vi "FPGA cRIOMain_v9.vi"() -> ()   [LabVIEW 2019]
uses:
  TypeDefs/AO mode TabCtrl.ctl
  TypeDefs/SamplingModeEnum.ctl
  TypeDefs/AI_channelEnum.ctl
  <vilib>/Platform/TimedLoop/XDataNode/timing_clust.ctl
  <vilib>/Platform/TimedLoop/XDataNode/nitl_modes.ctl
  <vilib>/Platform/TimedLoop/XDataNode/wakeup.ctl
  <vilib>/rvi/Emulation/niFpgaGetClockAttributes.vi
  <vilib>/rvi/Emulation/niFpgaSctlEmulationGetInTimedLoop.vi
  <vilib>/rvi/Emulation/niFpgaEmulationReportErrorSimple.vi
  <vilib>/rvi/eio/common/nirviEmuTemplateMethod_errors.vi
  <vilib>/rvi/Emulation/niFpgaEmulationIsFPGAContextNoSignature.vi
  <vilib>/rvi/errors/niFpgaSetErrorForExecOnDevCompSimple.vi
  <vilib>/rvi/eio/common/nirviEmuReportErrorAndStop.vi
  <vilib>/rvi/DataTransferAndStorage/Container/Common/niFpgaContainerGetUniqueNameForEmu.vi
  <vilib>/rvi/FIFO/Fifo_Resource/nirvififoEmulationSetSize.vi
  <vilib>/rvi/FIFO/Fifo_Resource/nirviFifoEmulationQueueMgr.vi
  <instcachedir>/0/nirviFifoEmulationQueueMgr_E5CAEC123FF24DC58D834DCA3CDAA9B5.lvgen/nirviFifoEmulationQueueMgr_E5CAEC123FF24DC58D834DCA3CDAA9B5_000.vi
  <vilib>/rvi/FIFO/Fifo_Resource/nirvififoEmulationDetermineInputValidOut.vi
  <vilib>/rvi/FIFO/Fifo_Resource/nirvififoEmulationCreateLock.vi
  <vilib>/rvi/Emulation/niFpgaProcessEmulError.vi
  <vilib>/rvi/FIFO/Fifo_Resource/nirvififoEmulationObtainLock.vi
  <vilib>/rvi/FIFO/Fifo_Resource/nirvififoEmulationReleaseLock.vi
  <vilib>/rvi/occurrence/nirviWaitOnOccurrenceBase.vi
  <vilib>/rvi/errors/nirviReportUnexpectedCaseInternalError.vi
  <vilib>/rvi/errors/nirviReportUnexpectedCaseInternalError (U32).vi
  <vilib>/rvi/Emulation/niFpgaCriticalErrorInLSC.vi
  <instcachedir>/0/nirviFifoEmulationQueueMgr_E5CAEC123FF24DC58D834DCA3CDAA9B5.lvgen/nirviFifoEmulationQueueMgr_E5CAEC123FF24DC58D834DCA3CDAA9B5_006.vi
  <vilib>/Utility/error.llb/Clear Errors.vi
  <vilib>/rvi/Memory/Memory_Emulation/niFpgaMemoryEmulationCacheClearOnFirstRun.vi
  <vilib>/rvi/Memory/Memory_Emulation/nirvimemoryEmulationManagerCache_MakeExclusive.vi
  <vilib>/rvi/Memory/Memory_Emulation/niFpgaMemoryEmulationValidateCache.vi
  <vilib>/rvi/Memory/Memory_Emulation/nirvimemoryEmulationManagerCache_InsertValue.vi
  <vilib>/rvi/Memory/Memory_Emulation/nirvimemoryEmulationManagerCache_ReleaseExclusive.vi
  <vilib>/rvi/Memory/Memory_Emulation/nirvimemoryEmulationManagerCache_GetValue.vi
  <vilib>/rvi/Memory/Memory_Emulation/nirvimemoryEmulationManagerCache_SetValue.vi
  <vilib>/rvi/Analysis/common/codeGenErrors/XNode/niFpgaXNodeCodeGenErrorHandle.vi
  <instcachedir>/0/nirviFifoEmulationQueueMgr_E5CAEC123FF24DC58D834DCA3CDAA9B5.lvgen/nirviFifoEmulationQueueMgr_E5CAEC123FF24DC58D834DCA3CDAA9B5_015.vi
  <vilib>/eio/EIONode/EIONode.xnode
  <vilib>/rvi/DataTransferAndStorage/Container/XNode/niFpgaContainer.xnode
  <vilib>/rvi/FIFO/Fifo_Resource/nirvififoEmulationWrite.vi
  <vilib>/rvi/FIFO/Fifo_Resource/nirvififoEmulationRead.vi
  <vilib>/rvi/DataTransferAndStorage/Register/Emulation/niFpgaRegisterEmulation.vi
  <vilib>/rvi/FXPMathLib/FxpMul/XNode/nifxpmath_Multiplier.xnode
  <vilib>/rvi/Analysis/measure/LMRsmpl/XNode/niFPGA Rational Resampler.xnode
  <vilib>/Platform/TimedLoop/XDataNode/XDataNode.xnode
  <vilib>/Platform/TimedLoop/XDataNode/XDNodeRunTimeDep.lvlib
  <vilib>/rvi/FXPMathLib/sim/FxpSim.dll
panel:
  out "FPGA AI-M DMA\nOverflow?":bool
  out "AI M-2 loop time-2 [ticks]":u32
  out "AI M loop time [ticks]":u32
  out "FPGA AI DMA\nOverflow?":bool
  out "AI Processing\nLoop Rate to high?":bool
  in  "AI Process Time [ticks]":u32=125
  in  "Select Channel":T1
  out "Unable to\nsample at desired\nSample Rate?":bool
  out "Processing Loop time [ticks]":u32
  in  "Sampling Mode":T2
  in  "AO mode":T3
  in  "AO Out [V]":fxp<+/-,18,5> format="%#.6g"
  in  "AO enable?":bool
  out "AI In [V]":fxp<+/-,25,5> format="%#.6g"
  out "FPGA AO DMA\nOverflow?":bool
  out "Int. Output":fxp<+/-,20,5> format="%.17g"
  out "Raw AI Input":fxp<+/-,25,5> format="%.21g"
  in  "Sample Time [ticks]":u32=125
  out "AO Loop time [ticks]":u32
  out "AI Loop time [ticks]":u32
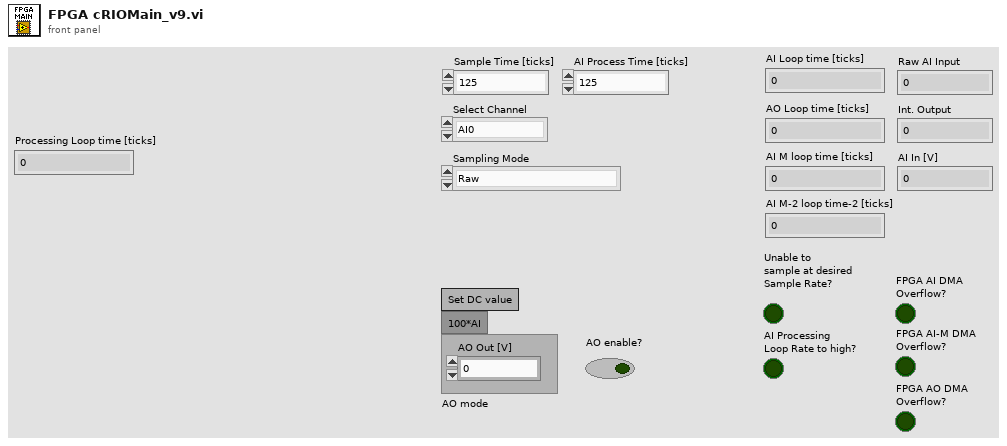
[diagram p1: front panel]
types:
  T1 = typedef "AI_channelEnum.ctl" = enum16{"AI0", "AI1", "AI2", "AI3"}
  T2 = typedef "SamplingModeEnum.ctl" = enum16{"Raw", "M64 (ReSpl)", "M128 (ReSpl)", "4pt MA (AI) + M64 (ReSpl)", "LPF (Proc.)", "4pt MA (AI) + LPF (Proc.)", "4pt MA (Proc.) + LPF (Proc.)"}
  T3 = typedef "AO mode TabCtrl.ctl" = enum32{"Set DC value", "100*AI"}
  T4 = typedef "XDNodeRunTimeDep.lvlib/timing_clust.ctl" = cluster{"Expected End [f-1]":u64, "Actual End [f-1]":u64, "Finished Late? [f-1]":bool, "Expected End [i-1]":u64, "Actual End [i-1]":u64, "Finished Late? [i-1]":bool, "Expected Start [i]":u64, "Actual Start [i]":u64, "Expected Start [f]":u64, "Actual Start [f]":u64, "Source Name":string, "Structure Name":string, "Period":i64, "Deadline":i64, "Offset":i64, "Start":i64, "Priority":i32, "Timeout":i32, "Mode":T5, "Wakeup Reason":T6, "Error":errorcluster, "Source Type":string, "Secondary Source Type":string, "Global End Time":u64, "Global Start Time":u64, "Frame Duration":u64, "Iteration Duration":u64, "Assigned CPU":i32, "I/O Scan Engine Mode":u32}
  T5 = typedef "XDNodeRunTimeDep.lvlib/nitl_modes.ctl" = enum32{"No Change", "Process missed periods, maintain original phase", "Discard missed periods, maintain original phase", "Process missed periods, ignore original phase", "Discard missed periods, ignore original phase"}
  T6 = typedef "XDNodeRunTimeDep.lvlib/wakeup.ctl" = enum32{"Normal", "Aborted", "Asynchronous wakeup", "Timing source error", "Timed loop error", "Timeout"}
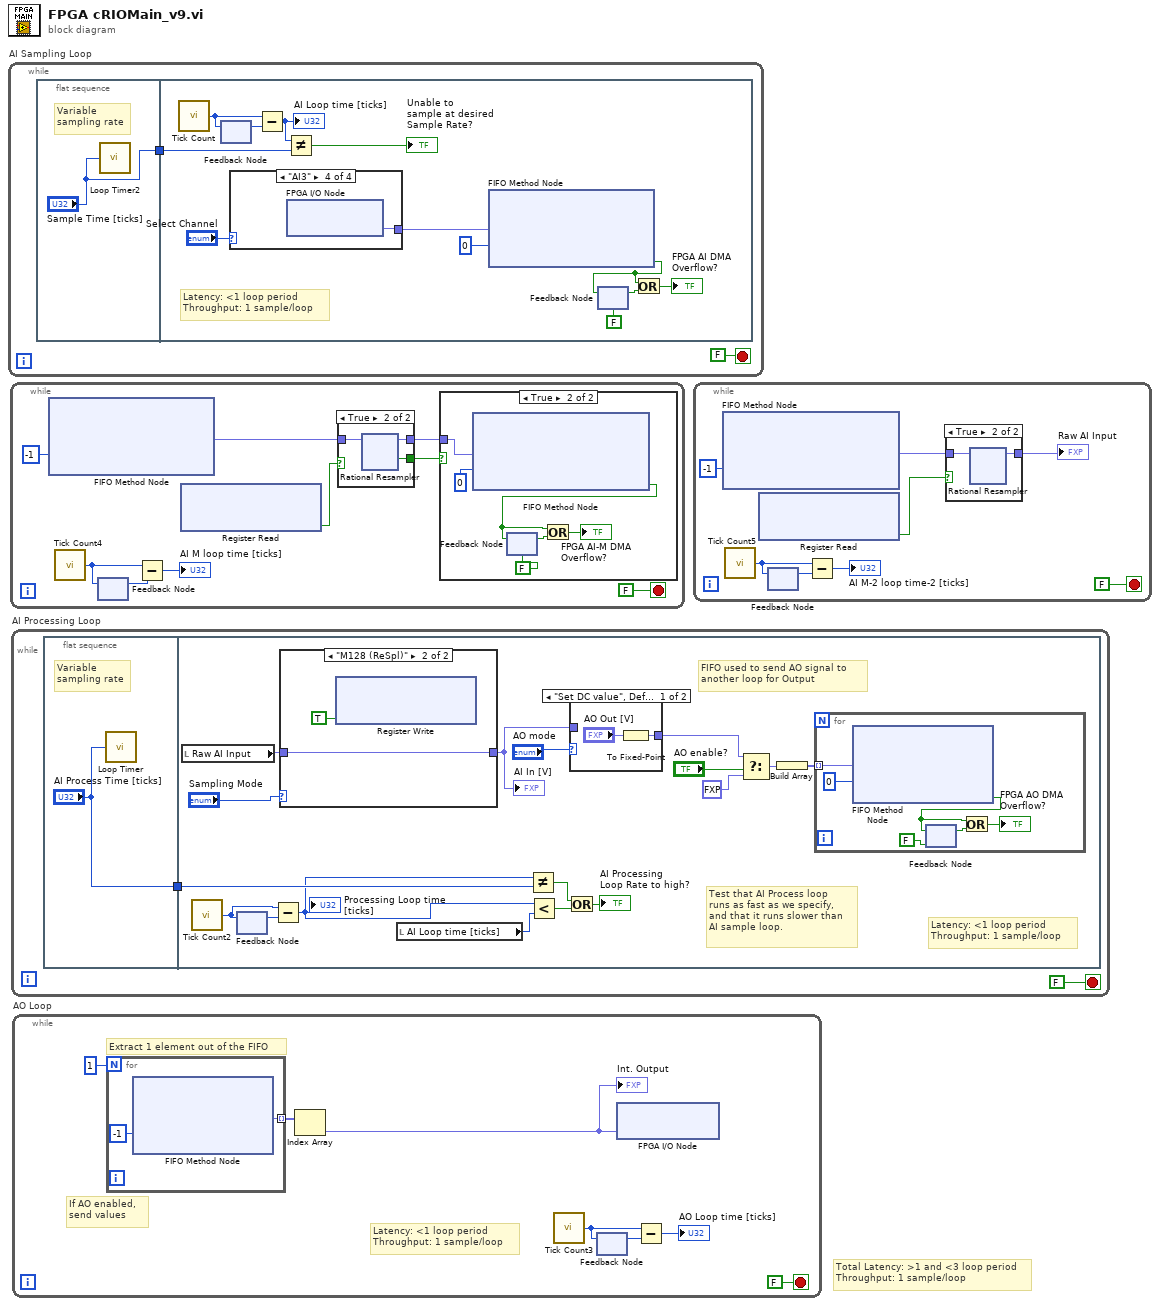
[diagram p0: block diagram]
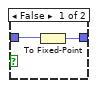
[diagram p2: hidden frame]
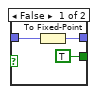
[diagram p4: hidden frame]
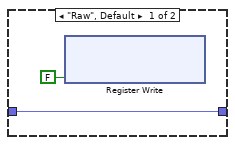
[diagram p5: hidden frame]
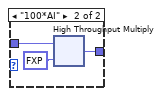
[diagram p6: hidden frame]
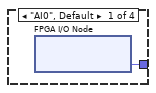
[diagram p7: hidden frame]
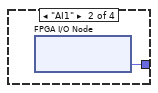
[diagram p8: hidden frame]
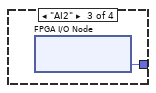
[diagram p9: hidden frame]
diagram:
  # "Total Latency: >1 and <3 loop period\nThroughput: 1 sample/loop"
  n1 = while "AI Sampling Loop" {
    stop <- FALSE stop-if-true
    n2 = flat-sequence {
      tunnel: ["Sample Time [ticks]"] -> w1
      tunnel: w1 -> [w12]
      frame #0 {
        # "Variable\nsampling rate"
        n3 = call "Loop Timer2"("Count(Ticks)"="Sample Time [ticks]") -> ()  [unwired: 1 out]
      }
      frame #1 {
        # "Latency: <1 loop period\nThroughput: 1 sample/loop"
        n4 = call "Tick Count"() -> ("Tick Count(Ticks)"=w15:u32)
        n5 = feedback #1() -> (w14:u32)  [unwired: 1 in]
        n6 = feedback-in #1(w15) -> ()
        n7 = case shown="\"AI3\"" "Select Channel" {
          tunnel: [w16 w17 w18 w19] -> w4
          frame "AI0", Default {
            n8 = xnode "FPGA I/O Node"() -> ("Mod4/AI0"=w16:fxp<+/-,24,5>)  [unwired: 1 in, 1 out]
          }
          frame "AI1" {
            n9 = xnode "FPGA I/O Node"() -> ("Mod4/AI1"=w17:fxp<+/-,24,5>)  [unwired: 1 in, 1 out]
          }
          frame "AI2" {
            n10 = xnode "FPGA I/O Node"() -> ("Mod4/AI2"=w18:fxp<+/-,24,5>)  [unwired: 1 in, 1 out]
          }
          frame "AI3" {
            n11 = xnode "FPGA I/O Node"() -> ("Mod4/AI3"=w19:fxp<+/-,24,5>)  [unwired: 1 in, 1 out]
          }
        }
        n12 = Subtract(x=w15, y=w14) -> (x-y=w13:u32)
        "AI Loop time [ticks]" <- w13
        n13 = Not Equal?(x=w13, y=w12) -> (x != y?=→"Unable to\nsample at desired\nSample Rate?":bool)
        n14 = xnode ("FIFO Method Node")("Element"=w4, "Timeout"=0) -> ("Timed Out?"=w7:bool)  [unwired: 1 in, 1 out]
        n15 = feedback #2(FALSE ("Timed Out?")) -> (w9:bool)
        n16 = feedback-in #2(w7) -> ()
        n17 = Or(x=w7, y=w9) -> (x .or. y?=→"FPGA AI DMA\nOverflow?":bool)
      }
    }
  }
  n18 = while {
    stop <- FALSE stop-if-true
    n19 = xnode ("FIFO Method Node")("Timeout"=-1) -> ("Element"=w22:fxp<+/-,24,5>)  [unwired: 1 in, 2 out]
    n20 = call "Tick Count4"() -> ("Tick Count(Ticks)"=w26:u32)
    n21 = feedback #3() -> (w25:u32)  [unwired: 1 in]
    n22 = feedback-in #3(w26) -> ()
    n23 = Subtract(x=w26, y=w25) -> (x-y=→"AI M loop time [ticks]":u32)
    n24 = xnode ("Register Read")() -> ("Data"=w23:bool)  [unwired: 1 in, 1 out]
    n25 = case shown="True" w23 {
      tunnel: w22 -> [w36 w40]
      tunnel: [w37 w39] -> w21
      tunnel: [TRUE ("output valid") w38] -> w20
      frame False {
        n26 = To Fixed-Point(number=w36) -> (fixed-point=w37:fxp<+/-,25,5>)  [unwired: 1 in]
      }
      frame True {
        n27 = xnode "Rational Resampler"("input data"=w40) -> ("output data"=w39:fxp<+/-,25,5>, "output valid"=w38:bool)  [unwired: 1 out]
      }
    }
    n28 = case shown="True" w20 {
      tunnel: w21 -> [_ w34]
      frame False {
      }
      frame True {
        n29 = xnode ("FIFO Method Node")("Element"=w34, "Timeout"=0) -> ("Timed Out?"=w29:bool)  [unwired: 1 in, 1 out]
        n30 = feedback #4(FALSE ("Timed Out?")) -> (w32:bool)
        n31 = feedback-in #4(w29) -> ()
        n32 = Or(x=w29, y=w32) -> (x .or. y?=→"FPGA AI-M DMA\nOverflow?":bool)
      }
    }
  }
  n33 = while "AI Processing Loop" {
    stop <- FALSE stop-if-true
    n34 = flat-sequence {
      tunnel: ["AI Process Time [ticks]"] -> w75
      tunnel: w75 -> [w79]
      frame #0 {
        # "Variable\nsampling rate"
        n35 = call "Loop Timer"("Count(Ticks)"="AI Process Time [ticks]") -> ()  [unwired: 1 out]
      }
      frame #1 {
        # "Test that AI Process loop\nruns as fast as we specify,\nand that it runs slower than \nAI sample loop."
        # "Latency: <1 loop period\nThroughput: 1 sample/loop"
        # "FIFO used to send AO signal to \nanother loop for Output"
        n36 = local read "Raw AI Input"() -> (w83:fxp<+/-,25,5>)
        n37 = call "Tick Count2"() -> ("Tick Count(Ticks)"=w93:u32)
        n38 = feedback #5() -> (w94:u32)  [unwired: 1 in]
        n39 = feedback-in #5(w93) -> ()
        n40 = Subtract(x=w93, y=w94) -> (x-y=w78:u32)
        "Processing Loop time [ticks]" <- w78
        n41 = case shown="\"M128 (ReSpl)\"" "Sampling Mode" {
          tunnel: [w95 w97] -> w91
          tunnel: w83 -> [w95 w97]
          frame "Raw", Default {
            n42 = xnode ("Register Write")("Data"=FALSE) -> ()  [unwired: 1 in, 1 out]
          }
          frame "M128 (ReSpl)" {
            n43 = xnode ("Register Write")("Data"=TRUE) -> ()  [unwired: 1 in, 1 out]
          }
        }
        "AI In [V]" <- w91
        n44 = local read "AI Loop time [ticks]"() -> (w84:u32)
        n45 = Not Equal?(x=w78, y=w79) -> (x != y?=w81:bool)
        n46 = Less?(x=w78, y=w84) -> (x < y?=w80:bool)
        n47 = Or(x=w81, y=w80) -> (x .or. y?=→"AI Processing\nLoop Rate to high?":bool)
        n48 = case shown="\"Set DC value\", Default" "AO mode" {
          tunnel: [w100 w101] -> w88
          tunnel: w91 -> [_ w103]
          frame "Set DC value", Default {
            n49 = To Fixed-Point(number="AO Out [V]") -> (fixed-point=w100:fxp<+/-,20,5>)  [unwired: 1 in]
          }
          frame "100*AI" {
            n50 = xnode ("High Throughput Multiply")("x"=w103, "y"=fxp<+,5,7> 100.0) -> ("x*y"=w101:fxp<+/-,20,5>)
          }
        }
        n51 = Select(t=w88, s="AO enable?", f=fxp<+/-,20,5> 0.0) -> (s? t:f=w92:fxp<+/-,20,5>)
        n52 = Build Array(w92) -> (w87:fxp<+/-,20,5>[])
        n53 = for {
          tunnel: w87 -> [w104] mode=indexing
          n54 = xnode ("FIFO Method Node")("Element"=w104, "Timeout"=0) -> ("Timed Out?"=w105:bool)  [unwired: 1 in, 1 out]
          n55 = feedback-in #6(w105) -> ()
          n56 = feedback #6(FALSE ("Timed Out?")) -> (w108:bool)
          n57 = Or(x=w105, y=w108) -> (x .or. y?=→"FPGA AO DMA\nOverflow?":bool)
        }
      }
    }
  }
  n58 = while "AO Loop" {
    stop <- FALSE stop-if-true
    # "Latency: <1 loop period\nThroughput: 1 sample/loop"
    # "If AO enabled, \nsend values"
    # "Extract 1 element out of the FIFO"
    n59 = for {
      N: 1 -> [_]
      tunnel: [w118] -> w112 mode=indexing
      n60 = xnode ("FIFO Method Node")("Timeout"=-1) -> ("Element"=w118:fxp<+/-,20,5>)  [unwired: 1 in, 2 out]
    }
    n61 = Index Array(array=w112) -> (element=w110:fxp<+/-,20,5>)  [unwired: 1 in]
    "Int. Output" <- w110
    n62 = call "Tick Count3"() -> ("Tick Count(Ticks)"=w115:u32)
    n63 = feedback #7() -> (w114:u32)  [unwired: 1 in]
    n64 = feedback-in #7(w115) -> ()
    n65 = xnode "FPGA I/O Node"("Mod3/AO1"=w110) -> ()  [unwired: 1 in, 1 out]
    n66 = Subtract(x=w115, y=w114) -> (x-y=→"AO Loop time [ticks]":u32)
  }
  n67 = while {
    stop <- FALSE stop-if-true
    n68 = xnode ("FIFO Method Node")("Timeout"=-1) -> ("Element"=w124:fxp<+/-,25,5>)  [unwired: 1 in, 2 out]
    n69 = call "Tick Count5"() -> ("Tick Count(Ticks)"=w121:u32)
    n70 = xnode ("Register Read")() -> ("Data"=w125:bool)  [unwired: 1 in, 1 out]
    n71 = feedback #8() -> (w120:u32)  [unwired: 1 in]
    n72 = feedback-in #8(w121) -> ()
    n73 = Subtract(x=w121, y=w120) -> (x-y=→"AI M-2 loop time-2 [ticks]":u32)
    n74 = case shown="True" w125 {
      tunnel: [w128 w130] -> w123
      tunnel: w124 -> [w127 w129]
      frame False {
        n75 = To Fixed-Point(number=w127) -> (fixed-point=w128:fxp<+/-,25,5>)  [unwired: 1 in]
      }
      frame True {
        n76 = xnode "Rational Resampler"("input data"=w129) -> ("output data"=w130:fxp<+/-,25,5>)  [unwired: 2 out]
      }
    }
    "Raw AI Input" <- w123
  }
